vi "Manager1.vi"() -> ()   [LabVIEW 2018]
uses:
  <vilib>/DAQmx/read.llb/DAQmx Read (Digital Bool 1Line 1Point).vi
  <vilib>/DAQmx/write.llb/DAQmx Write (Digital Bool 1Line 1Point).vi
  <vilib>/DAQmx/miscellaneous.llb/DAQmx Fill In Error Info.vi
panel:
  in  "stop":bool
  out "data":bool
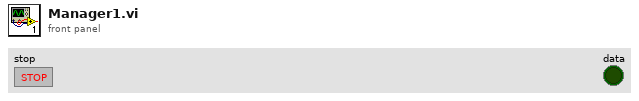
[diagram p1: front panel]
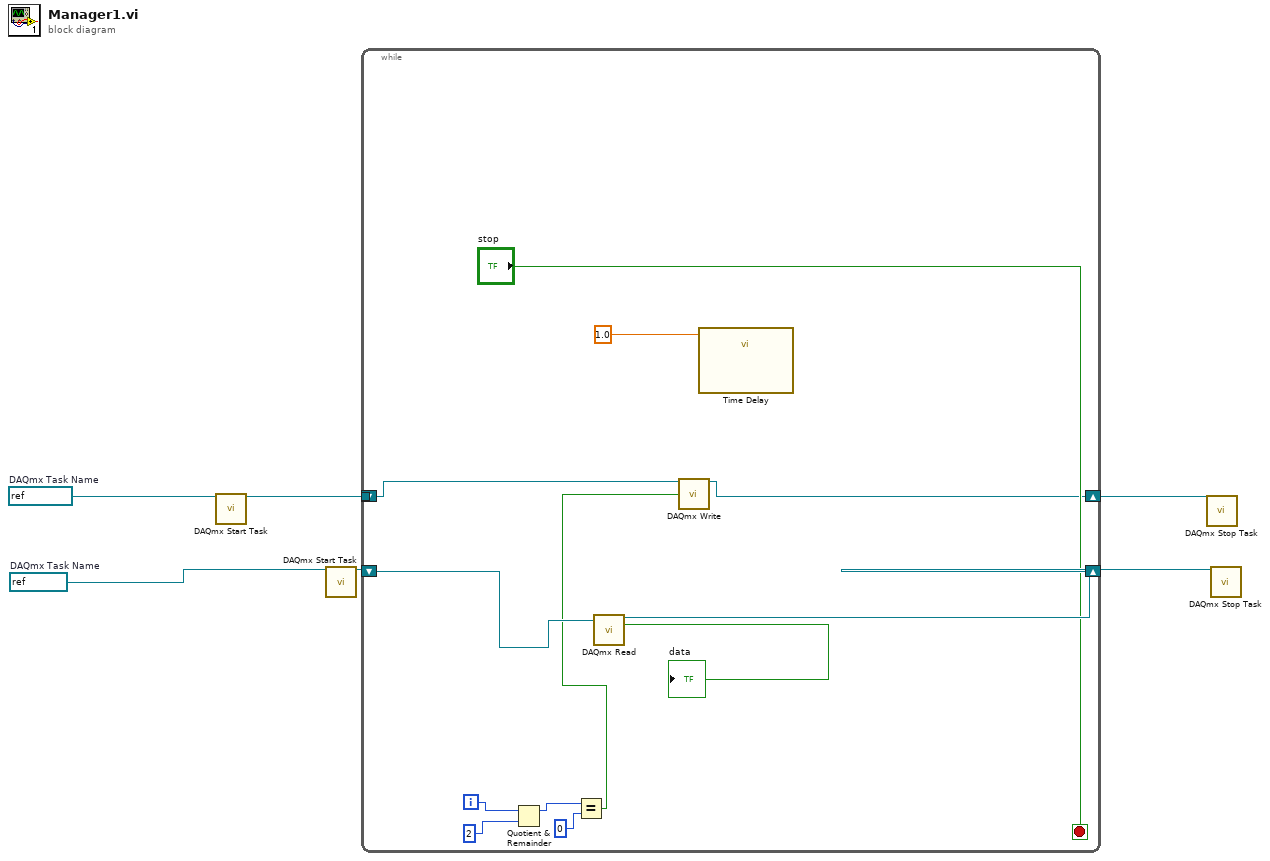
[diagram p0: block diagram]
diagram:
  w5 = refnum<k21> "TEST2"  # DAQmx Task Name
  w6 = refnum<k21> "TEST21"  # DAQmx Task Name
  n1 = call <vilib>:"DAQmx Start Task.vi"("task/channels in"=w6) -> ("task out"=w1:refnum<k21>)  [unwired: 13 in, 1 out]
  n2 = call <vilib>:"DAQmx Start Task.vi"("task/channels in"=w5) -> ("task out"=w4:refnum<k21>)  [unwired: 13 in, 1 out]
  n3 = while {
    shift-right: [w9] -> w2
    shift-left: w1 -> [w8]
    shift-right: [w17] -> w3
    shift-left: w4 -> [w18]
    tunnel: [w8] -> _
    i -> [w13]
    stop <- "stop" stop-if-true
    n4 = Quotient & Remainder(x=w13, y=2) -> (x-y*floor(x/y)=w11:i32)  [unwired: 1 out]
    n5 = Equal?(x=w11, y=0) -> (x = y?=w7:bool)
    n6 = call-poly <vilib>:"DAQmx Read.vi"("task/channels in"=w18) -> ("task out"=w17:refnum<k21>, "data"=→"data":bool)  [unwired: 12 in, 1 out]
    n7 = call-poly <vilib>:"DAQmx Write.vi"("task/channels in"=w8, "data"=w7) -> ("task out"=w9:refnum<k21>)  [unwired: 11 in, 2 out]
    n8 = call "Time Delay"("Delay Time (s)"=1.0) -> ()  [unwired: 10 in, 1 out]
  }
  n9 = call <vilib>:"DAQmx Stop Task.vi"("task/channels in"=w2) -> ()  [unwired: 13 in, 2 out]
  n10 = call <vilib>:"DAQmx Stop Task.vi"("task/channels in"=w3) -> ()  [unwired: 13 in, 2 out]
